vi "Main Interface.vi"() -> ()   [LabVIEW 2015]
uses:
  CRD/Data/tCRD Data.lvclass
  Reusable/Xctls/Configurable Buffer/Configurable Buffer.xctl
  <vilib>/Utility/miscctls.llb/LVPositionTypeDef.ctl
  <vilib>/event_ctls.llb/eventvkey.ctl
  Devices/Alicat/Session Based/Data/MC/MC Data.lvclass
  Devices/Alicat/Session Based/Data/M/M data.lvclass
  Reusable/General/Math Utilities.lvlib
  <vilib>/Analysis/NI_AALBase.lvlib
  <vilib>/Analysis/1siggen.llb/Ramp Pattern by Delta.vi
  Reusable/CRDS/Data/Cell/CRDS Cell Data.lvclass
  Devices/Airmar/Data/Airmar Data.lvclass
  FPGA/Rate.ctl
  Reusable/CRDS/Data/Cell/extparam.ctl
panel:
  in  "writeTaus":bool
  out "LastZero":timestamp caption="Last Zero" format="%<%H:%M:%S%2u\n%m/%d>T"
  out "filtLastSw":timestamp caption="Last Zero" format="%<%H:%M:%S%2u\n%m/%d>T"
  in  "nephtremains":dbl caption="Next Switch (s)"
  in  "tSwitch":dbl caption="Next Switch (s)"
  in  "newFile":bool
  in  "restart":bool
  in  "SyncTime":bool
  out "Zeroing?":bool
  in  "writeRDs":bool
  in  "mainTab":enum32{"Main", "Control", "Auxilary", "wsData"}(tab)
  out "rd":dbl[][](graph)
  out "tau (us)":sgl
  out "Data In":sgl(graph)
  out "eRD":dbl[](graph)
  out "rData":cluster{"RH (%)":sgl, "T deg(C)":sgl} caption="Rotronic Data" {"T deg(C)" format="%6.2f"; "RH (%)" format="%6.2f"}
  in  "Invert?":bool
  out "Drive Space (Mb)":u32
  in  "Qpurge (lpm)":cluster{"Sample":sgl, "Zero":sgl} {"Zero" min=0 step=0.01 format="%.2g"; "Sample" min=0 step=0.01 format="%.2g"}
  out "Alicat Data":T1
  in  "Laser Off (us)":u32=16
  in  "# to Coadd":u8=16 min=1 max=50 step=1
  in  "Bank 3":bool
  in  "Bank 2":bool
  in  "Bank 1":bool
  in  "Heater Power":bool
  out "Neph Aux Data":T2
  out "Neph Data":T3
  in  "Power":bool
  in  "Blower":u8
  in  "Autozero Mode":enum16{"Manual", "Auto"}(ring)
  in  "Manual Zero":bool
  in  "Rate":T4=10 items=["1 MHz"=20, "2 MHz"=10, "2.5 MHz"=8, "5 MHz"=4, "10 MHz"=2, "20MHz"=1]
  in  "Sample Time (us)":u16=100
  in  "Delay (us)":u16=16
  in  "Frequency (Hz)":dbl
  in  "cycle?":bool
  in  "Sample (s)":dbl
  in  "Zero (s)":dbl
  in  "Servo Position (deg)":cluster{u32, u32}(slide)={806, 2337} scale=500.0..2500.0
  in  "Lock":bool=TRUE
  in  "Zero State":bool
  out "vData":cluster{"RH (%)":sgl, "T deg(C)":sgl} caption="Vaisala Data" {"T deg(C)" format="%6.2f"; "RH (%)" format="%6.2f"}
  out "GGA":T5 caption="Airmar GPS Data" {"UTC" format="%<%H:%M:%S%2u>T"}
  out "mda":T6 caption="Airmar Met Data"
  out "Path":path
  out "File Size":u32
  out "u":sgl format="%.2f"
  out "extParam":T7={"Tau"=nan, "Tau0cor"=nan, "ext"=nan, "extCorr"=nan, "stdevTau"=nan, "eTau"=nan, "taucorr"=nan, "Tau0"=nan, "max"=nan} caption="Extinction Parameters" {"Tau0" format="%#.2f"; "taucorr" format="%#.2f"; "eTau" format="%#.2f"; "stdevTau" format="%#.2f"; "extCorr" format="%.2f"; "ext" format="%#.2f"; "Tau0cor" format="%#.2f"; "Tau" format="%#.2f"}
  out "Tv":cluster{"Val":dbl[], "time":timestamp}(xcontrol)
  out "RHv":cluster{"Val":dbl[], "time":timestamp}(xcontrol)
  out "Anemometer":cluster{"Val":dbl[], "time":timestamp}(xcontrol)
  out "windSpeed":cluster{"Val":dbl[], "time":timestamp}(xcontrol)
  out "Tmet":cluster{"Val":dbl[], "time":timestamp}(xcontrol)
  out "RHmet":cluster{"Val":dbl[], "time":timestamp}(xcontrol)
  out "windDir":cluster{"Val":dbl[], "time":timestamp}(xcontrol)
  out "Version":string
  in  "Save":bool
  out "time":timestamp format="%<%H:%M:%S%2u>T"
  # "CRD Zero"
  # "Neph State"
  # "OPEN PATH DATA"
  # "CONTROL"
  # "Open Path CRD Control"
  # "Laser/Sample Control"
  # "Servo"
  # "Nephelometer"
  # "Fan Control"
  # "AUXILARY DATA"
  # "AIRMAR DATA"
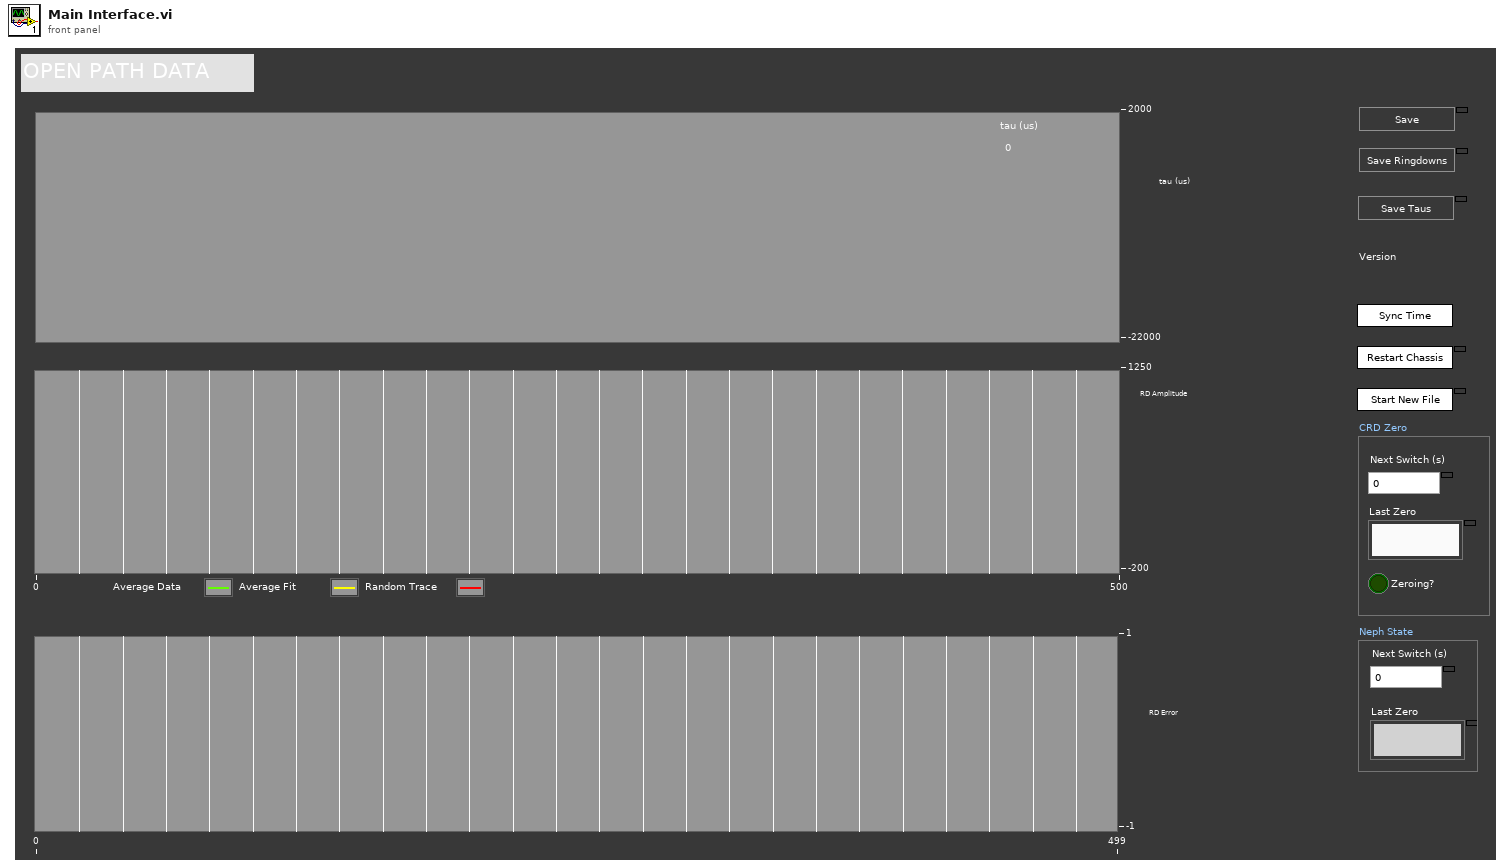
[diagram p1: front panel]
types:
  T1 = cluster{"P (mb)":dbl, "T (degC)":dbl, "Q (lpm)":dbl, "Q (slpm)":dbl, "Qsp":dbl}
  T2 = cluster{"Sensitivity":dbl, "Pressure":dbl, "Tsample":dbl, "Tinlet":dbl, "RH":dbl, "Vlamp":dbl, "Ilamp":dbl}
  T3 = cluster{"Mode":enum16{"Normal", "Zero", "Blank"}, "Scatter Mode":enum16{"Total Scatter", "Back Scatter"}, "Cblue":dbl, "Cgreen":dbl, "Cred":dbl, "Cback,blue":dbl, "Cback,green":dbl, "Cback,red":dbl}
  T4 = typedef "Rate.ctl" = u8
  T5 = cluster{"UTC":timestamp, "Latitude":dbl, "N/S":enum8{"North", "South"}, "Longitude":dbl, "E/W":enum8{"East", "West"}, "GPS Quality":enum16{"Fix not available or invalid", "GPS SPS Mode, fix valid", "Differential GPS, SPS Mode, fix valid", "GPS PPS Mode, fix valid", "Real Time Kinematic", "Float RTK", "Estimated (dead reckoning) Mode", "Manual Input Mode", "Simulator Mode"}, "Number of Satellites":u8, "MSL Altitude":dbl}
  T6 = cluster{"Pressure":dbl, "T (degC)":dbl, "RH (%)":dbl, "Td (degC)":dbl, "True Wind Direction":dbl, "Magnetic Wind Direction":dbl, "Wind Speed (m/s)":dbl}
  T7 = typedef "extparam.ctl" = cluster{"Tau":sgl, "Tau0cor":sgl, "ext":sgl, "extCorr":sgl, "stdevTau":sgl, "eTau":sgl, "taucorr":sgl, "Tau0":sgl, "max":sgl}
  T8 = enum32{"Invalid", "Standard", "Closed", "Hidden", "Minimized", "Maximized"}
  T9 = typedef "LVPositionTypeDef.ctl" = cluster{"Left":i32, "Top":i32}
  T10 = typedef "eventvkey.ctl" = enum16{"ASCII", "Enter", "Return", "Shift", "Ctrl", "Alt", "Cmd", "Opt", "Caps", "NumLock", "Clear", "Break", "Up", "Down", "Left", "Right", "Insert", "Delete", "Home", "End", "PageUp", "PageDown", "Escape", "Help", "Pause", "ScrollLock", "F1", "F2", "F3", "F4", "F5", "F6", "F7", "F8", "F9", "F10", "F11", "F12", "F13", "F14", "F15", "F16", "F17", "F18", "F19", "F20", "F21", "F22", "F23", "F24", "Play", "VolumeUp", "VolumeDown", "Mute", "Two Byte Char"}
  T11 = enum8{"Enabled", "Disabled", "Disabled and Grayed Out"}
  T12 = cluster{"Barometric Pressure":dbl, "Temperature":dbl, "Relative Humidity":dbl, "Dew Point":dbl, "True Wind Direction":dbl, "Magnetic Wind Direction":dbl, "Wind Speed":dbl}
  T13 = cluster{"Accessors:P":sgl, "Accessors:T":sgl, "Accessors:Q":sgl, "Accessors:Q0":sgl, "Accessors:Qsp":sgl}
  T14 = cluster{"[0]":dbl, "[1]":dbl, "[2]":dbl, "[3]":dbl, "[4]":dbl, "[5]":dbl, "[6]":dbl, "[7]":dbl}
  T15 = cluster{"[0]":dbl, "[1]":dbl, "[2]":dbl, "[3]":dbl, "[4]":dbl, "[5]":dbl, "[6]":dbl}
  T16 = cluster{"Array of Single[0]":sgl, "Array of Single[1]":sgl}
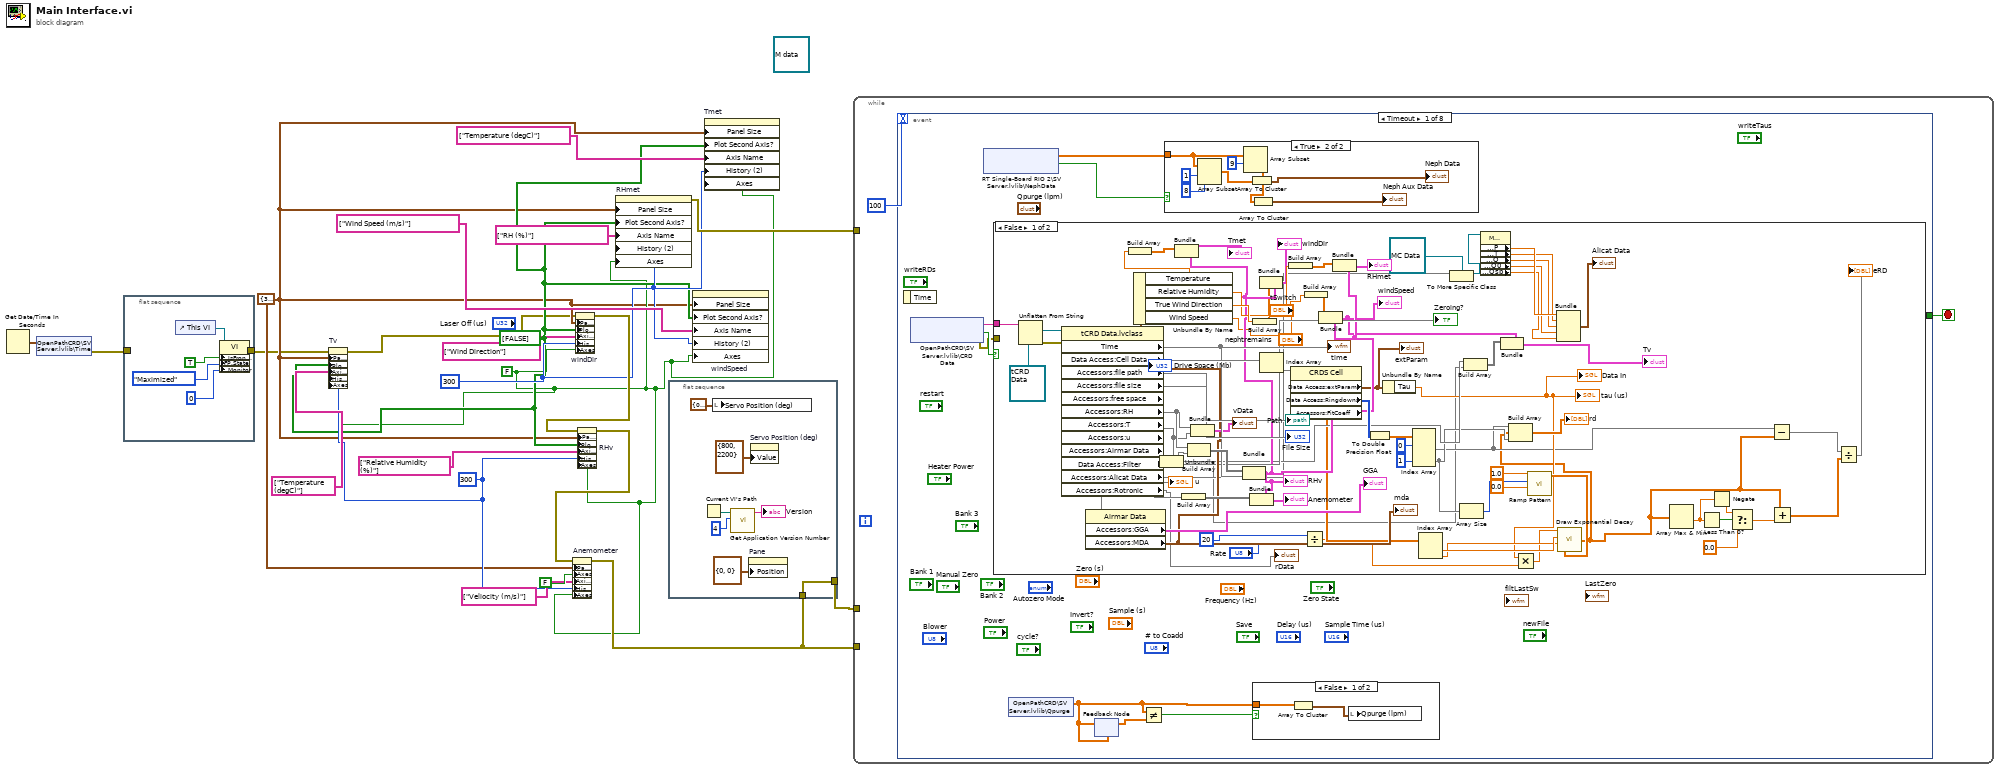
[diagram p0: block diagram]
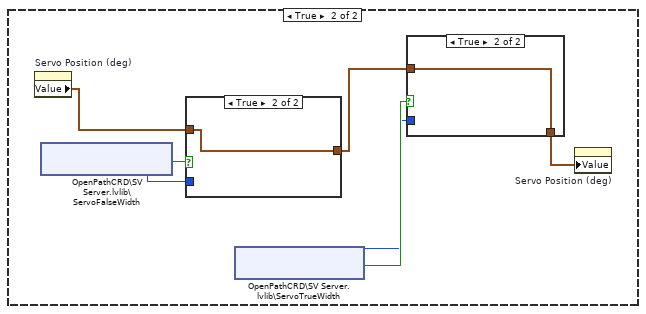
[diagram p4: hidden frame]
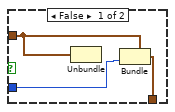
[diagram p5: hidden frame]
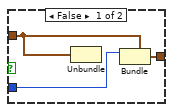
[diagram p6: hidden frame]
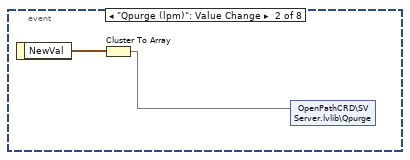
[diagram p7: hidden frame]
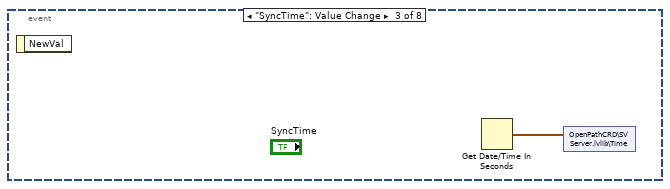
[diagram p8: hidden frame]
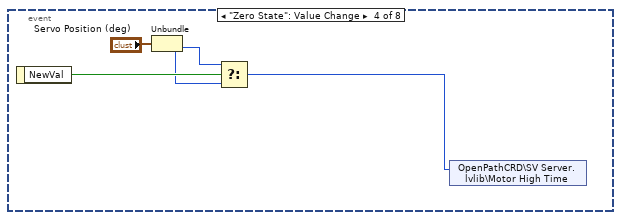
[diagram p9: hidden frame]
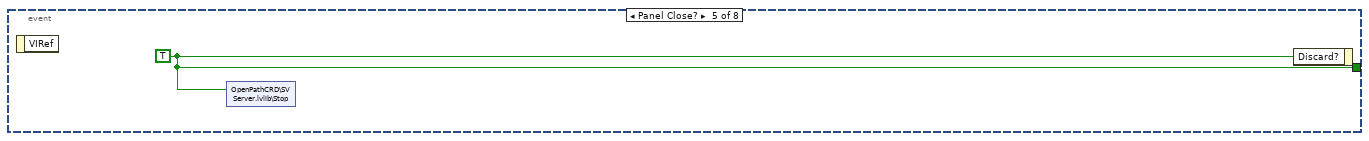
[diagram p10: hidden frame]
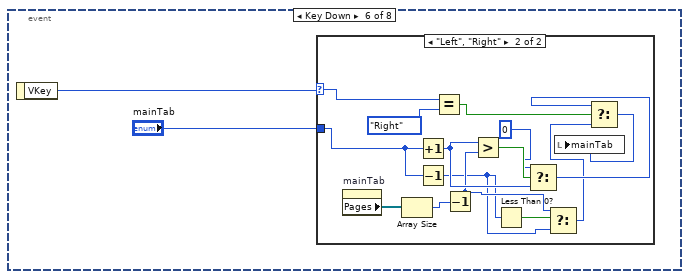
[diagram p11: hidden frame]
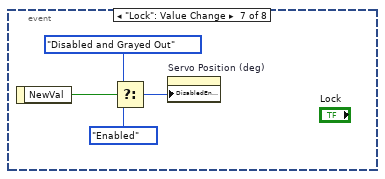
[diagram p13: hidden frame]
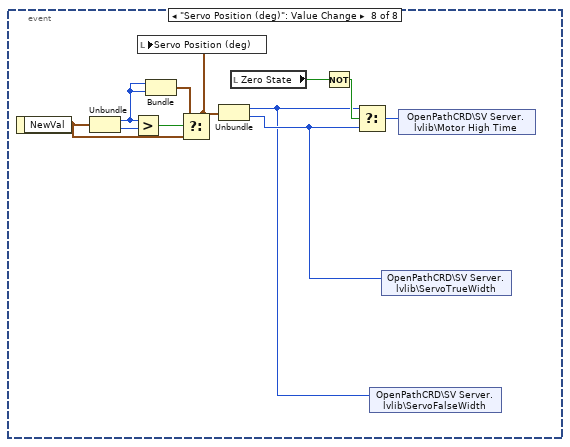
[diagram p14: hidden frame]
diagram:
  (unwired) refnum<class "M data.lvclass"> refnum ("M Data")
  w6 = FALSE ("Two Axes?")
  w5 = cluster{"Height":i16, "Width":i16} {"Height"=325, "Width"=525} ("Panel Size")
  w7 = bool[] [FALSE] ("Plot Second Axis?")
  w11 = 300 ("History")
  w8 = 300 ("History")
  n1 = Get Date/Time In Seconds() -> (seconds since 1Jan1904=w3:timestamp)
  n2 = shared-variable "OpenPathCRD\\SV Server.lvlib\\Time"(w3) -> (error out=w1:errorcluster)  [unwired: 1 in]
  n3 = flat-sequence {
    tunnel: [w23] -> w4
    tunnel: w1 -> [_]
    frame #0 {
      n4 = control-ref of="This VI"() -> (w27:refnum<vi>)
      n5 = property class="VI"(reference=w27, "Front Panel.IsFrontmost"=TRUE ("Front Panel Window:Is Frontmost"), "FP.State"=T8."Maximized" ("Front Panel Window:State"), "FP.Monitor"=u16 0 ("Front Panel Window:Monitor")) -> (error out=w23:errorcluster)  [unwired: 1 in, 1 out]
    }
  }
  n6 = property on="Tv" class="Configurable Buffer (strict)"(error in=w4, "Panel Size"=w5, "Plot Second Axis?"=w7, "Axis Name"=string[] ["Temperature (degC)"], "History (2)"=w8, "Axes"=w6) -> (error out=w2:errorcluster)  [unwired: 1 in, 1 out]
  n7 = property on="windDir" class="Configurable Buffer (strict)"(error in=w2, "Panel Size"=w5, "Plot Second Axis?"=w7, "Axis Name"=string[] ["Wind Direction"], "History (2)"=w11, "Axes"=w6) -> (error out=w17:errorcluster)  [unwired: 1 in, 1 out]
  n8 = property on="RHv" class="Configurable Buffer (strict)"(error in=w17, "Panel Size"=w5, "Plot Second Axis?"=w7, "Axis Name"=string[] ["Relative Humidity (%)"], "History (2)"=w8, "Axes"=w6) -> (error out=w22:errorcluster)  [unwired: 1 in, 1 out]
  n9 = property on="Anemometer" class="Configurable Buffer (strict)"(error in=w22, "Panel Size"=w5, "Axes"=FALSE ("Two Axes?"), "Axis Name"=string[] ["Veliocity (m/s)"], "History (2)"=w8, "Axes"=w6) -> (error out=w10:errorcluster)  [unwired: 1 in, 1 out]
  n10 = property on="RHmet" class="Configurable Buffer (strict)"("Panel Size"=w5, "Plot Second Axis?"=w7, "Axis Name"=string[] ["RH (%)"], "History (2)"=w11, "Axes"=w6) -> (error out=w15:errorcluster)  [unwired: 2 in, 1 out]
  n11 = flat-sequence {
    tunnel: [w28] -> w14
    tunnel: w10 -> [w28]
    frame #0 {
      n12 = Current VI's Path() -> (path=w31:path)
      n13 = local write "Servo Position (deg)"(cluster{dbl, dbl} {0.0, 90.0} ("Servo Position (deg)")) -> ()
      n14 = call "Get Application Version Number.vi"("Number to Strip"=4, "Initial Path"=w31) -> ("Version"=→"Version":string)  [unwired: 8 in, 1 out]
      n15 = property on="Pane" class="Pane"("Position"=T9 {"Left"=0, "Top"=0}) -> ()  [unwired: 2 in, 2 out]
      n16 = property on="Servo Position (deg)" class="Slide (strict)"("Value"=cluster{u32, u32} {800, 2200} ("Servo Position (deg)")) -> ()  [unwired: 2 in, 2 out]
    }
  }
  n17 = property on="windSpeed" class="Configurable Buffer (strict)"("Panel Size"=w5, "Plot Second Axis?"=w7, "Axis Name"=string[] ["Wind Speed (m/s)"], "History (2)"=w11, "Axes"=w6) -> ()  [unwired: 2 in, 2 out]
  n18 = property on="Tmet" class="Configurable Buffer (strict)"("Panel Size"=w5, "Plot Second Axis?"=w7, "Axis Name"=string[] ["Temperature (degC)"], "History (2)"=w11, "Axes"=w6) -> ()  [unwired: 2 in, 2 out]
  n19 = while {
    tunnel: w10 -> [_]
    tunnel: w15 -> [_]
    tunnel: w14 -> [_]
    stop <- w36 stop-if-true
    n20 = event shown="[0] Timeout" {
      selector: _ -> [_ _ _ _ _ _ _ _]
      dyn-events: _ -> [_ _ _ _ _ _ _ _]
      timeout: 100 -> [_ _ _ _ _ _ _ _]
      tunnel: [_ _ _ _ w154 _ _ _] -> w36
      event Timeout {
        n21 = event-data() -> ()  [unwired: 1 in, 1 out]
        n22 = shared-variable "OpenPathCRD\\SV Server.lvlib\\CRD Data"() -> (w44:string, error out=w37:errorcluster, w43:bool)  [unwired: 2 in]
        n23 = shared-variable "RT Single-Board RIO 2\\SV Server.lvlib\\NephData"() -> (w41:dbl[], w42:bool)  [unwired: 2 in, 1 out]
        n24 = case shown="False" w43 {
          tunnel: w44 -> [w130 _]
          tunnel: w37 -> [_ _]
          frame False {
            n25 = Unflatten From String(type=refnum<class "tCRD Data.lvclass"> refnum ("tCRD Data"), binary string=w130) -> (value=w129:refnum<class "tCRD Data.lvclass">, error out=w128:errorcluster)  [unwired: 3 in, 1 out]
            n26 = property class="tCRD Data.lvclass" props=["Time", "Data Access:Cell Data", "Accessors:file path", "Accessors:file size", "Accessors:free space", "Accessors:RH", "Accessors:T", "Accessors:u", "Accessors:Airmar Data", "Data Access:Filter", "Accessors:Alicat Data", "Accessors:Rotronic"](reference=w129, error in=w128) -> ("Time"=w117, "Data Access:Cell Data"=w127, "Accessors:file path"=→"Path", "Accessors:file size"=→"File Size", "Accessors:RH"=w111, "Accessors:T"=w95, "Accessors:u"=w116, "Accessors:Airmar Data"=w113, "Data Access:Filter"=→"Zeroing?", "Accessors:Alicat Data"=w90, "Accessors:Rotronic"=w57)  [unwired: 3 out]
            "time" <- w117
            "u" <- w116
            "rData" <- w57
            n27 = property class="Airmar Data"(reference=w113) -> ("Accessors:GGA"=→"GGA":T5, "Accessors:MDA"=w109:T12)  [unwired: 1 in, 2 out]
            "mda" <- w109
            n28 = Unbundle By Name(w109) -> ("Temperature"=w101:dbl, "Relative Humidity"=w107:dbl, "True Wind Direction"=w108:dbl, "Wind Speed"=w98:dbl)
            n29 = Build Array(w101) -> (w100:dbl[])
            n30 = Unbundle(w57) -> (w56, w55)
            n31 = Build Array(w116) -> (w115:void[])
            n32 = Build Array(w111, w56) -> (w118:void[])
            n33 = Bundle("Accessors:RH"=w111, "Accessors:T"=w95) -> (→"vData":cluster{"Accessors:RH":void, "Accessors:T":void})  [unwired: 1 in]
            n34 = Bundle(w118, "Time"=w117) -> (w99:cluster{void[], "Time":void})  [unwired: 1 in]
            "RHv" <- w99
            n35 = Bundle(cluster=w99, w100) -> (→"Tmet":cluster{void[], "Time":void})  [unwired: 1 in]
            n36 = Bundle(cluster=w99, w115) -> (→"Anemometer":cluster{void[], "Time":void})  [unwired: 1 in]
            n37 = Build Array(w108) -> (w96:dbl[])
            n38 = Bundle(cluster=w99, w96) -> (→"windDir":cluster{void[], "Time":void})  [unwired: 1 in]
            n39 = Index Array(array=w127) -> (element=w126)  [unwired: 1 in]
            n40 = Build Array(w107) -> (w106:dbl[])
            n41 = property class="CRDS Cell"(reference=w126) -> ("Data Access:extParam"=w82:T7, "Data Access:Ringdowns"=w120:i16[][], "Accessors:FitCoeff"=w81:dbl[])  [unwired: 1 in, 2 out]
            "extParam" <- w82
            n42 = Divide(x=20, y="Rate") -> (x/y=w69:dbl)
            n43 = Build Array(w98) -> (w97:dbl[])
            n44 = Bundle(cluster=w99, w97) -> (w93:cluster{void[], "Time":void})  [unwired: 1 in]
            "windSpeed" <- w93
            n45 = Bundle(cluster=w99, w106) -> (→"RHmet":cluster{void[], "Time":void})  [unwired: 1 in]
            n46 = To Double Precision Float(number=w120) -> (double precision float=w119:dbl[][])
            n47 = Unbundle By Name(w82) -> ("Tau"=w70:sgl)
            "Data In" <- w70
            "tau (us)" <- w70
            n48 = Index Array(array=w119, index (row) #1=0 ("index (row)"), index (row) #2=1 ("index (row)")) -> (element #1=w62:dbl[], element #2=w76:dbl[])  [unwired: 2 in]
            n49 = Index Array(array=w81) -> (element #1=w80:dbl, element #2=w79:dbl)  [unwired: 2 in]
            n50 = To More Specific Class(target class=refnum<class "MC Data.lvclass"> refnum ("MC Data"), reference=w90) -> (specific class reference=w89:refnum<class "MC Data.lvclass">)  [unwired: 1 in, 1 out]
            n51 = Array Size(array=w76) -> (size(s)=w75:i32)
            n52 = Build Array(w95, w55) -> (w94:void[])
            n53 = property class="MC Data"(reference=w89) -> ("Accessors:P"=w88:sgl, "Accessors:T"=w87:sgl, "Accessors:Q"=w86:sgl, "Accessors:Q0"=w85:sgl, "Accessors:Qsp"=w84:sgl)  [unwired: 1 in, 2 out]
            n54 = Bundle(cluster=w93, w94) -> (→"Tv":cluster{void[], "Time":void})  [unwired: 1 in]
            n55 = Multiply(x=w70, y=w69) -> (x*y=w68:dbl)
            n56 = call-poly <vilib>:"Ramp Pattern.vi"("start"=0.0, "end"=w75, "delta"=1.0) -> ("Ramp Pattern"=w78:dbl[])  [unwired: 6 in, 2 out]
            n57 = Bundle("Accessors:P"=w88, "Accessors:T"=w87, "Accessors:Q"=w86, "Accessors:Q0"=w85, "Accessors:Qsp"=w84) -> (→"Alicat Data":T13)  [unwired: 1 in]
            n58 = call "Draw Exponential Decay.vi"("time"=w78, "B"=w79, "A"=w80, "tau"=w68) -> ("ExponentialOut"=w58:dbl[])
            n59 = Build Array(w62, w58, w76) -> (→"rd":dbl[][])
            n60 = Array Max & Min(array=w58) -> (min value=w60:dbl)  [unwired: 3 out]
            n61 = Less Than 0?(x=w60) -> (x < 0?=w67:bool)
            n62 = Negate(x=w60) -> (-x=w59:dbl)
            n63 = Select(t=w59, s=w67, f=0.0) -> (s? t:f=w61:dbl)
            n64 = Subtract(x=w62, y=w58) -> (x-y=w65:dbl[])
            n65 = Add(x=w58, y=w61) -> (x+y=w63:dbl[])
            n66 = Divide(x=w65, y=w63) -> (x/y=→"eRD":dbl[])
          }
          frame True {
            n67 = property on="Servo Position (deg)" class="Slide (strict)"() -> ("Value"=w136:cluster{u32, u32})  [unwired: 2 in, 2 out]
            n68 = shared-variable "OpenPathCRD\\SV Server.lvlib\\ServoFalseWidth"() -> (w135:u32, w137:bool)  [unwired: 2 in, 1 out]
            n69 = case shown="True" w137 {
              tunnel: w136 -> [w144 w145]
              tunnel: w135 -> [w143 _]
              tunnel: [w142 w145] -> w134
              frame False {
                n70 = Unbundle(w144) -> ()  [unwired: 2 out]
                n71 = Bundle(cluster=w144, w143) -> (w142:cluster{u32, u32})  [unwired: 1 in]
              }
              frame True {
              }
            }
            n72 = shared-variable "OpenPathCRD\\SV Server.lvlib\\ServoTrueWidth"() -> (w132:u32, w133:bool)  [unwired: 2 in, 1 out]
            n73 = case shown="True" w133 {
              tunnel: w134 -> [w140 w141]
              tunnel: w132 -> [w139 _]
              tunnel: [w138 w141] -> w131
              frame False {
                n74 = Unbundle(w140) -> ()  [unwired: 2 out]
                n75 = Bundle(cluster=w140, w139) -> (w138:cluster{u32, u32})  [unwired: 1 in]
              }
              frame True {
              }
            }
            n76 = property on="Servo Position (deg)" class="Slide (strict)"("Value"=w131) -> ()  [unwired: 2 in, 2 out]
          }
        }
        n77 = shared-variable "OpenPathCRD\\SV Server.lvlib\\Qpurge"() -> (w38:sgl[])  [unwired: 1 in, 1 out]
        n78 = feedback-in #1(w38) -> ()
        n79 = feedback #1(w38) -> (w40:sgl[])
        n80 = Not Equal?(x=w38, y=w40) -> (x != y?=w39:bool)
        n81 = case shown="True" w42 {
          tunnel: w41 -> [_ w50]
          frame False {
          }
          frame True {
            n82 = Array Subset(array=w50, index=1, length=8) -> (w52:dbl[])
            n83 = Array Subset(array=w50, index=9) -> (w48:dbl[])  [unwired: 1 in]
            n84 = Array To Cluster(array=w52) -> (cluster=→"Neph Data":T14)
            n85 = Array To Cluster(array=w48) -> (cluster=→"Neph Aux Data":T15)
          }
        }
        n86 = case shown="False" w39 {
          tunnel: w38 -> [w46 _]
          frame False {
            n87 = Array To Cluster(array=w46) -> (cluster=w45:T16)
            n88 = local write "Qpurge (lpm)"(w45) -> ()
          }
          frame True {
          }
        }
      }
      event "Qpurge (lpm)": Value Change {
        n89 = event-data() -> ("NewVal"=w147:cluster{"Sample":sgl, "Zero":sgl})  [unwired: 1 in]
        n90 = Cluster To Array(cluster=w147) -> (array=w146:sgl[])
        n91 = shared-variable "OpenPathCRD\\SV Server.lvlib\\Qpurge"(w146) -> ()  [unwired: 1 in, 1 out]
      }
      event "SyncTime": Value Change {
        n92 = event-data() -> ()  [unwired: 1 in, 1 out]
        n93 = Get Date/Time In Seconds() -> (seconds since 1Jan1904=w148:timestamp)
        n94 = shared-variable "OpenPathCRD\\SV Server.lvlib\\Time"(w148) -> ()  [unwired: 1 in, 1 out]
      }
      event "Zero State": Value Change {
        n95 = event-data() -> ("NewVal"=w153:bool)  [unwired: 1 in]
        n96 = Unbundle("Servo Position (deg)") -> (w151:u32, w150:u32)
        n97 = Select(t=w150, s=w153, f=w151) -> (s? t:f=w149:u32)
        n98 = shared-variable "OpenPathCRD\\SV Server.lvlib\\Motor High Time"(w149) -> ()  [unwired: 1 in, 1 out]
      }
      event Panel Close? {
        w154 = TRUE ("Discard?")
        n99 = event-data() -> ()  [unwired: 1 in, 1 out]
        n100 = shared-variable "OpenPathCRD\\SV Server.lvlib\\Stop"(w154) -> ()  [unwired: 1 in, 1 out]
        n101 = event-data("Discard?"=w154) -> ()  [unwired: 1 in, 1 out]
      }
      event Key Down {
        n102 = event-data() -> ("VKey"=w156:T10)  [unwired: 1 in]
        n103 = case shown="\"Left\", \"Right\"" w156 {
          selector: w156 -> [_ w170]
          tunnel: "mainTab" -> [_ w162]
          frame "ASCII", Default {
          }
          frame "Left", "Right" {
            n104 = property on="mainTab" class="TabCtl (strict)"() -> ("Pages"=w171:refnum<vi>[])  [unwired: 2 in, 2 out]
            n105 = Array Size(array=w171) -> (size(s)=w167:i32)
            n106 = Increment(x=w162) -> (x+1=w165:enum32{"Main", "Control", "Auxilary", "wsData"})
            n107 = Decrement(x=w162) -> (x-1=w159:enum32{"Main", "Control", "Auxilary", "wsData"})
            n108 = Equal?(x=w170, y=eventvkey."Right") -> (x = y?=w168:bool)
            n109 = Decrement(x=w167) -> (x-1=w160:i32)
            n110 = Greater?(x=w165, y=w160) -> (0:w166:bool)
            n111 = Less Than 0?(x=w159) -> (x < 0?=w161:bool)
            n112 = Select(t=0, s=w166, f=w165) -> (s? t:f=w163:u32)
            n113 = Select(t=w160, s=w161, f=w159) -> (s? t:f=w158:u32)
            n114 = Select(t=w163, s=w168, f=w158) -> (s? t:f=w157:u32)
            n115 = local write "mainTab"(w157) -> ()
          }
        }
      }
      event "Lock": Value Change {
        n116 = event-data() -> ("NewVal"=w175:bool)  [unwired: 1 in]
        n117 = Select(t=T11."Disabled and Grayed Out" ("Disabled"), s=w175, f=T11."Enabled" ("Disabled")) -> (s? t:f=w172:T11)
        n118 = property on="Servo Position (deg)" class="Slide (strict)"("DisabledEnum"=w172) -> ()  [unwired: 2 in, 2 out]
      }
      event "Servo Position (deg)": Value Change {
        n119 = event-data() -> ("NewVal"=w184:cluster{u32, u32})  [unwired: 1 in]
        n120 = Unbundle(w184) -> (w183:u32, w186:u32)
        n121 = Greater?(x=w183, y=w186) -> (0:w185:bool)
        n122 = Bundle(w183, w183) -> (w182:cluster{u32, u32})  [unwired: 1 in]
        n123 = Select(t=w182, s=w185, f=w184) -> (s? t:f=w181:cluster{u32, u32})
        n124 = local write "Servo Position (deg)"(w181) -> ()
        n125 = Unbundle(w181) -> (w176:u32, w177:u32)
        n126 = local read "Zero State"() -> (w179:bool)
        n127 = Not(x=w179) -> (.not. x?=w178:bool)
        n128 = Select(t=w176, s=w178, f=w177) -> (s? t:f=w180:u32)
        n129 = shared-variable "OpenPathCRD\\SV Server.lvlib\\ServoFalseWidth"(w176) -> ()  [unwired: 1 in, 1 out]
        n130 = shared-variable "OpenPathCRD\\SV Server.lvlib\\ServoTrueWidth"(w177) -> ()  [unwired: 1 in, 1 out]
        n131 = shared-variable "OpenPathCRD\\SV Server.lvlib\\Motor High Time"(w180) -> ()  [unwired: 1 in, 1 out]
      }
    }
  }
